vi "Stop Core.vi"(10 "final error code":i32, 11 "DMM Driver in":refnum<class "DMM Driver.lvclass">) -> (3 "DMM Driver out":refnum<class "DMM Driver.lvclass">)   [LabVIEW 2020, in "DMM Driver.lvclass"]
doc: "(<B>Filename</B>: Actor Framework.lvlib:Actor.lvclass:Stop Core.vi)\n\nDefines what the actor does before it stops. Use the <B>final error code</B> input to determine whether the actor shut down in response to an error.\n\nBy default, this method does nothing. A descendant class may override it to define behavior, such as shutting down any processes the actor initiated in its override of the Actor Core method."
uses:
  DMM Driver.lvclass
  <vilib>/ActorFramework/Actor/Actor.lvclass
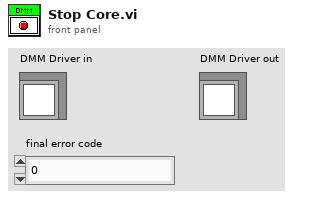
[diagram p1: front panel]
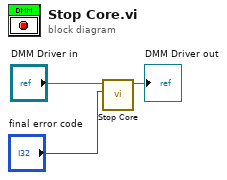
[diagram p0: block diagram]
diagram:
  n1 = call-parent "Stop Core.vi"("final error code"="final error code", "Actor in"="DMM Driver in") -> ("Actor out"=→"DMM Driver out":refnum<class "DMM Driver.lvclass">)  [unwired: 9 in]
